vi "Write Sequence Parameters.vi"(8 "error in (no error)":errorcluster, 10 "Sequence Parameters":cluster{"Buffer Size":dbl, "Sample Rate":dbl}, 11 "ChannelConfig in":refnum<class "ChannelConfig.lvclass">) -> (0 "error out":errorcluster, 3 "ChannelConfig out":refnum<class "ChannelConfig.lvclass">)   [LabVIEW 2015, in "Channel.lvlib" / "ChannelConfig.lvclass"]
uses:
  ChannelConfig.lvclass
  ChannelConfig.lvclass/ChannelConfig.ctl
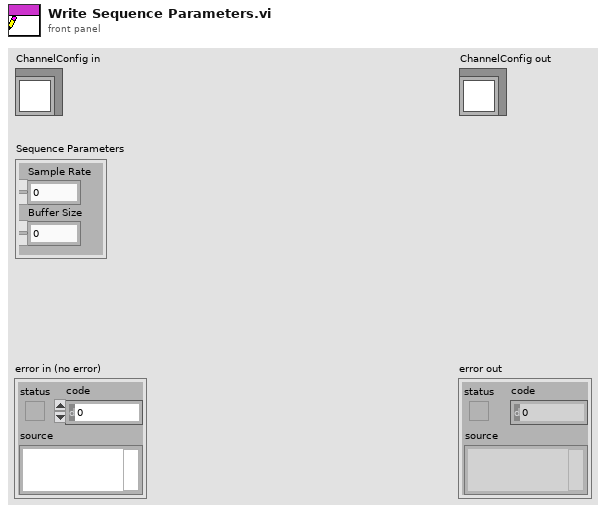
[diagram p1: front panel]
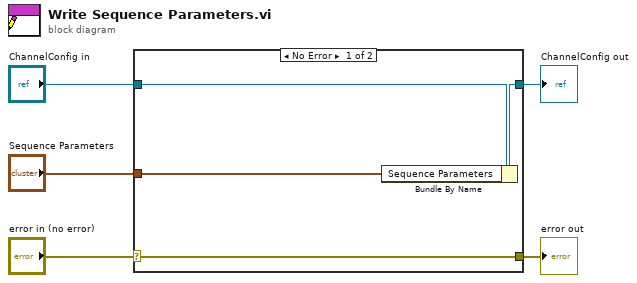
[diagram p0: block diagram]
diagram:
  n1 = case shown="No Error" "error in (no error)" {
    selector: "error in (no error)" -> [w9 w10]
    tunnel: [w9 w10] -> w4
    tunnel: [w7 w11] -> w2
    tunnel: "ChannelConfig in" -> [w8 w11]
    tunnel: "Sequence Parameters" -> [w6 _]
    frame No Error {
      n2 = Bundle By Name(cluster=w8, "Sequence Parameters"=w6) -> (w7:refnum<class "ChannelConfig.lvclass">)
    }
    frame Error {
    }
  }
  "error out" <- w4
  "ChannelConfig out" <- w2
